vi "IT6000C Output DC Volts.vi"() -> ()   [LabVIEW 2015]
doc: "This example shows how to configure the instrument's output voltage level, over current protection, and over voltage protection. The actual voltage level and actual current level are returned as well as whether over voltage protection (OVP) or over current protection (OCP) has been tripped."
uses:
  <instrlib>/IT6000C/IT6000C.lvlib
panel:
  in  "CURRent Limit (0.0 A)":dbl
  in  "Enable OCP (T: Enable)":bool=TRUE
  in  "Enable OVP (T: Enable)":bool=TRUE
  in  "Serial Configuration":T1={"Baud Rate"=9600, "Parity"=0, "Data Bits"=8, "Stop Bits"=10, "Flow Control"=0} {"Flow Control" items=["None", "XON/XOFF", "RTS/CTS", "XON/XOFF & RTS/CTS", "DTR/DSR", "XON/XOFF & DTR/DSR"]; "Stop Bits" items=["1.0"=10, "1.5"=15, "2.0"=20]; "Data Bits" items=["7"=7, "8"=8]; "Parity" items=["None", "Odd", "Even", "Mark", "Space"]; "Baud Rate" items=["300"=300, "600"=600, "1200"=1200, "2400"=2400, "4800"=4800, "9600"=9600, "19200"=19200]}
  in  "Stop Output":bool
  in  "OVP LEVEL (0V)":dbl format="%.2f"
  out "Actual Current Limit (A)":dbl format="%.2f"
  out "Actual Voltage Level (V)":dbl format="%.2f"
  in  "Voltage Level (0.0 V)":dbl format="%.2f"
  in  "OCP LEVEL (0A)":dbl format="%.2f"
  in  "VISA resource name":refnum<visa-resource-name>
  # "(c) 2014 <Enter Company Name Here>.  ALL RIGHTS RESERVED."
  # "Over Voltage Protection"
  # "Over Current Protection"
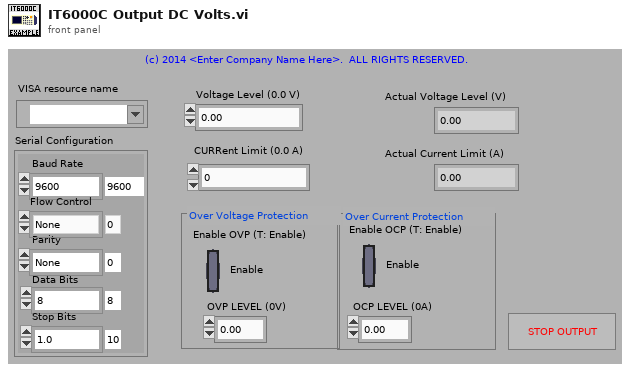
[diagram p1: front panel]
types:
  T1 = cluster{"Baud Rate":u32, "Parity":u16, "Data Bits":u16, "Stop Bits":u16, "Flow Control":u16}
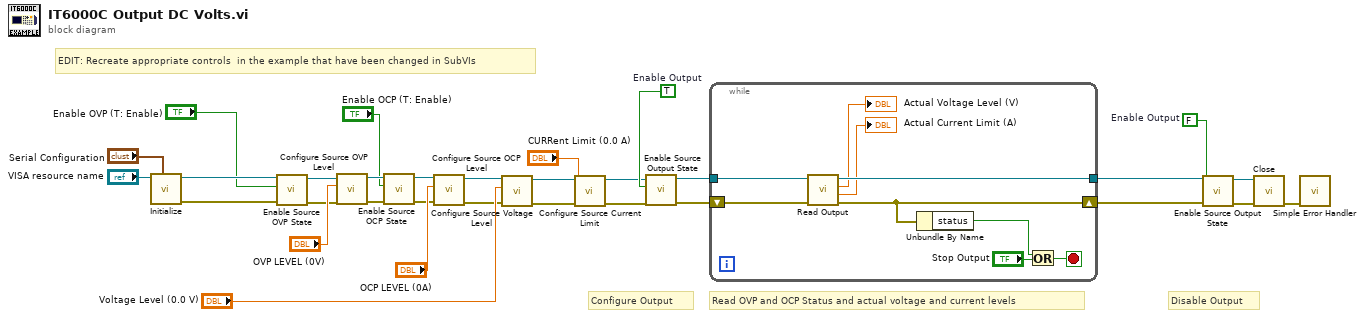
[diagram p0: block diagram]
diagram:
  w23 = FALSE  # Enable Output
  w19 = TRUE  # Enable Output
  # "EDIT: Recreate appropriate controls  in the example that have been changed in SubVIs"
  # "Disable Output"
  # "Read OVP and OCP Status and actual voltage and current levels"
  # "Configure Output"
  n1 = call <instrlib>:"Initialize.vi"("Serial Configuration"="Serial Configuration", "VISA resource name"="VISA resource name") -> ("error out"=w15:errorcluster, "VISA resource name out"=w16:refnum<visa-resource-name>)  [unwired: 8 in]
  n2 = call <instrlib>:"Enable Source OVP State.vi"("error in (no error)"=w15, "Enable(True)"="Enable OVP (T: Enable)", "VISA resource name"=w16) -> ("error out"=w18:errorcluster, "VISA resource name out"=w17:refnum<visa-resource-name>)  [unwired: 7 in]
  n3 = call <instrlib>:"Configure Source OVP Level.vi"("error in (no error)"=w18, "Value(0)"="OVP LEVEL (0V)", "VISA resource name"=w17) -> ("error out"=w13:errorcluster, "VISA resource name out"=w12:refnum<visa-resource-name>)  [unwired: 7 in]
  n4 = call <instrlib>:"Enable Source OCP State.vi"("error in (no error)"=w13, "Enable(True)"="Enable OCP (T: Enable)", "VISA resource name"=w12) -> ("error out"=w10:errorcluster, "VISA resource name out"=w11:refnum<visa-resource-name>)  [unwired: 7 in]
  n5 = call <instrlib>:"Configure Source OCP Level.vi"("error in (no error)"=w10, "Value(0)"="OCP LEVEL (0A)", "VISA resource name"=w11) -> ("error out"=w6:errorcluster, "VISA resource name out"=w8:refnum<visa-resource-name>)  [unwired: 7 in]
  n6 = call <instrlib>:"Configure Source Voltage Level.vi"("error in (no error)"=w6, "Value(0)"="Voltage Level (0.0 V)", "VISA resource name"=w8) -> ("error out"=w4:errorcluster, "VISA resource name out"=w5:refnum<visa-resource-name>)  [unwired: 7 in]
  n7 = call <instrlib>:"Configure Source Current Limit.vi"("error in (no error)"=w4, "Value(0)"="CURRent Limit (0.0 A)", "VISA resource name"=w5) -> ("error out"=w2:errorcluster, "VISA resource name out"=w3:refnum<visa-resource-name>)  [unwired: 7 in]
  n8 = call <instrlib>:"Enable Source Output State.vi"("error in (no error)"=w2, "Enable(True)"=w19, "VISA resource name"=w3) -> ("error out"=w29:errorcluster, "VISA resource name out"=w30:refnum<visa-resource-name>)  [unwired: 7 in]
  n9 = while {
    tunnel: w30 -> [w39]
    tunnel: [w40] -> w28
    shift-right: [w33] -> w27
    shift-left: w29 -> [w38]
    stop <- w35 stop-if-true
    n10 = call <instrlib>:"Read Output.vi"("error in (no error)"=w38, "VISA resource name"=w39) -> ("error out"=w33:errorcluster, "Actual Current Level (A)"=→"Actual Current Limit (A)":dbl, "Actual Voltage Level (V)"=→"Actual Voltage Level (V)":dbl, "VISA resource name out"=w40:refnum<visa-resource-name>)  [unwired: 6 in]
    n11 = Unbundle By Name(w33) -> ("status"=w32:bool)
    n12 = Or(x=w32, y="Stop Output") -> (x .or. y?=w35:bool)
  }
  n13 = call <instrlib>:"Enable Source Output State.vi"("error in (no error)"=w27, "Enable(True)"=w23, "VISA resource name"=w28) -> ("error out"=w25:errorcluster, "VISA resource name out"=w26:refnum<visa-resource-name>)  [unwired: 7 in]
  n14 = call <instrlib>:"Close.vi"("error in (no error)"=w25, "VISA resource name"=w26) -> ("error out"=w22:errorcluster)  [unwired: 9 in]
  n15 = call <vilib>:"Simple Error Handler.vi"("error in (no error)"=w22) -> ()  [unwired: 4 in, 5 out]
